vi "generateJobGUID.vi"(8 "error in (no error)":errorcluster, 11 "Job in":refnum<class "Job.lvclass">) -> (0 "error out":errorcluster, 3 "Job out":refnum<class "Job.lvclass">)   [LabVIEW 2013, in "openCronJob.lvlib" / "Job.lvclass"]
uses:
  Job.lvclass
  Job.lvclass/Job.ctl
  <vilib>/LabVIEW Open Source Project/Unicity/RandomStringGenerator/RandomStringGenerator.lvclass
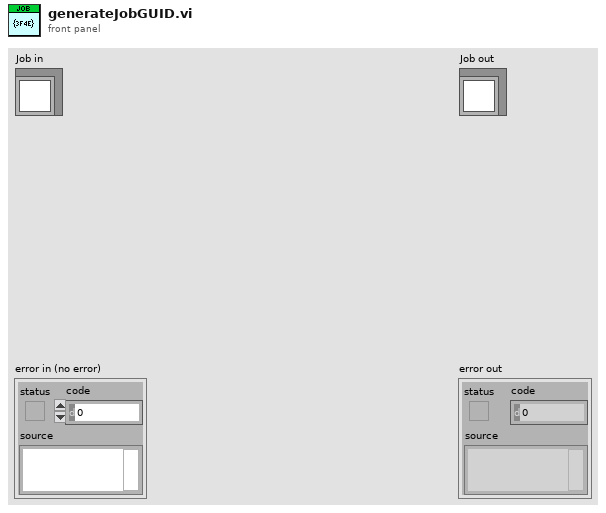
[diagram p1: front panel]
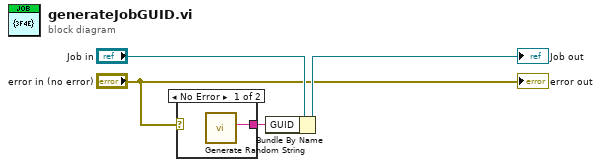
[diagram p0: block diagram]
diagram:
  n1 = case shown="No Error" "error in (no error)" {
    tunnel: [w5 _] -> w2
    frame No Error {
      n2 = call <vilib>:"Generate Random String.vi"() -> ("Random String"=w5:string)  [unwired: 11 in]
    }
    frame Error {
    }
  }
  n3 = Bundle By Name(cluster="Job in", "GUID"=w2) -> (→"Job out":refnum<class "Job.lvclass">)
  "error out" <- "error in (no error)"
